vi "Complex selector (array).vi"(10 "Domain (mag)":T1, 11 "Array (CDB)":cdb[](array[numeric])) -> (3 "Part (DBL)":dbl[](array[numeric]))   [LabVIEW 2020]
uses:
  Domain.ctl
  <vilib>/Analysis/NI_AALPro.lvlib
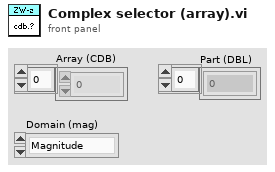
[diagram p1: front panel]
types:
  T1 = typedef "Domain.ctl" = enum16{"Magnitude", "Phase", "Phase unwrp", "Real", "Imaginary"}
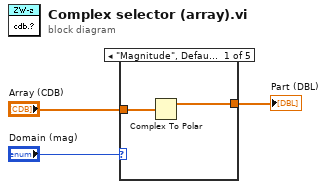
[diagram p0: block diagram]
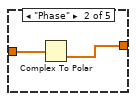
[diagram p2: hidden frame]
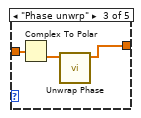
[diagram p3: hidden frame]
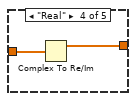
[diagram p4: hidden frame]
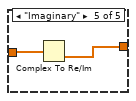
[diagram p5: hidden frame]
diagram:
  n1 = case shown="\"Magnitude\", Default" "Domain (mag)" {
    tunnel: "Array (CDB)" -> [w5 w7 w10 w12 w14]
    tunnel: [w4 w6 w8 w11 w13] -> w3
    frame "Magnitude", Default {
      n2 = Complex To Polar(r * e^(i*theta)=w5) -> (r=w4:dbl[])  [unwired: 1 out]
    }
    frame "Phase" {
      n3 = Complex To Polar(r * e^(i*theta)=w7) -> (theta=w6:dbl[])  [unwired: 1 out]
    }
    frame "Phase unwrp" {
      n4 = Complex To Polar(r * e^(i*theta)=w10) -> (theta=w9:dbl[])  [unwired: 1 out]
      n5 = call <vilib>:"Unwrap Phase.vi"("Phase"=w9) -> ("Unwrapped Phase"=w8:dbl[])  [unwired: 9 in, 1 out]
    }
    frame "Real" {
      n6 = Complex To Re/Im(x + iy=w12) -> (x=w11:dbl[])  [unwired: 1 out]
    }
    frame "Imaginary" {
      n7 = Complex To Re/Im(x + iy=w14) -> (y=w13:dbl[])  [unwired: 1 out]
    }
  }
  "Part (DBL)" <- w3
